vi "Stop Live Mode.vi"(8 "error in (no error)":errorcluster, 11 "Photometrics Camera in":refnum<class "Photometrics Camera.lvclass">) -> (0 "error out":errorcluster, 3 "Photometrics Camera out":refnum<class "Photometrics Camera.lvclass">)   [LabVIEW 2023, in "Photometrics Camera.lvlib" / "Photometrics Camera.lvclass"]
uses:
  Photometrics Camera.lvclass
  Photometrics Camera.lvclass/Photometrics Camera.ctl
  fb183b99-018c-4626-9964-c2e6b7479c68.vi
  <userlib>/TPM LabVIEW adapter/Camera/Camera.lvclass
  Camera/Camera.lvclass
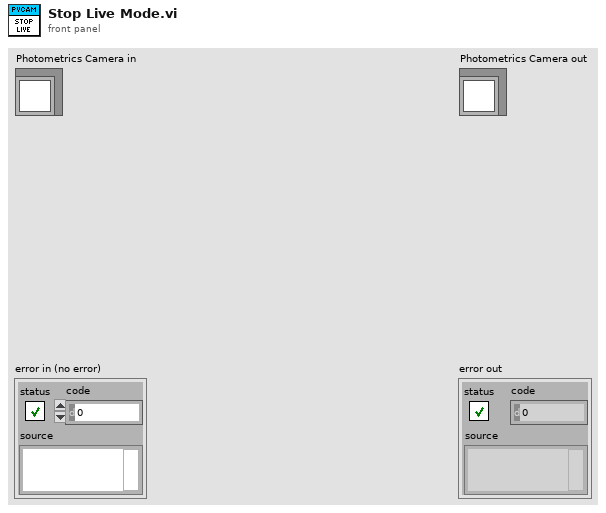
[diagram p1: front panel]
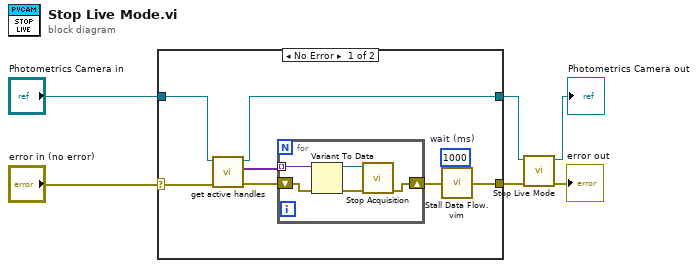
[diagram p0: block diagram]
diagram:
  n1 = case shown="No Error" "error in (no error)" {
    selector: "error in (no error)" -> [w13 w21]
    tunnel: [w8 w21] -> w3
    tunnel: "Photometrics Camera in" -> [w12 w20]
    tunnel: [w11 w20] -> w1
    frame No Error {
      w7 = u32 1000  # wait (ms)
      n2 = call-dynamic "get active handles.vi"("error in (no error)"=w13, "Camera in"=w12) -> ("error out"=w14:errorcluster, "Handles"=w10:variant[], "Camera out"=w11:refnum<class "Photometrics Camera.lvclass">)  [unwired: 5 in, 2 out]
      n3 = for {
        tunnel: w10 -> [w17] mode=indexing
        shift-right: [w19] -> w9
        shift-left: w14 -> [w18]
        n4 = Variant To Data(error in=w18, Variant=w17) -> (data=w16:refnum<class "Camera.lvclass">, error out=w15:errorcluster)  [unwired: 1 in]
        n5 = call <userlib>:"Stop Acquisition.vi"("error in (no error)"=w15, "Camera in"=w16) -> ("error out"=w19:errorcluster)  [unwired: 8 in, 1 out]
      }
      n6 = call "Stall Data Flow.vim"("value in"=w9, "milliseconds to wait"=w7) -> ("value out"=w8:errorcluster)  [unwired: 1 out]
    }
    frame Error {
    }
  }
  n7 = call-parent "Stop Live Mode.vi"("error in (no error)"=w3, "Camera in"=w1) -> ("error out"=→"error out":errorcluster, "Camera out"=→"Photometrics Camera out":refnum<class "Photometrics Camera.lvclass">)  [unwired: 8 in]
